vi "pmtProjectorGating2.vi"() -> ()   [LabVIEW 2012]
doc: "I. Description:\nThis example demonstrates how to output a retriggerable waveform using the internal output of a counter for the sample clock.\n\nII. Instructions for Running:\n1. Select the Physical Channel to correspond to where your signal is output on the DAQ device.\n2. Enter the Minimum and Maximum Voltage Ranges\n3. Enter the Counter Channel to generate a pulse train for the sample clock\n4. Select the Clock Source to be the Internal Output of the counter chosen in the previous step. If you cannot see this option, right-click on the control, choose I/O Name Filtering …, and select \"Include Advanced Terminals\" \n5. Select the Trigger Source to correspond to the terminal on which the trigger will be received\n6. Select the Trigger Edge to be rising or falling\n7. Specify the Desired Frequency of the output Waveform\n8. Enter the Waveform Information. See the documentation of the Waveform Buffer Generation SubVI for information on each parameter.\n\nIII. Block Diagram Steps:\nSteps: \n1. Create an Analog Output Voltage channel and a Counter Output Frequency channel.\n2. Use the Waveform Buffer subVI to create the waveform. \n3. Call the DAQmx Timing (Implicit) VI which sets the sample clock rate based on the frequency of the pulse train, and set the sample mode to finite. The number of Sample per Buffer corresponds to the number of samples per channel the counter output channel will produce. Set the DAQmx Timing (Sample Clock) VI to use the Internal Output of the counter as its Clock Source and set the sample mode to continuous.\n4. Call the DAQmx Start Trigger VI to set the Source and Trigger Edge. \n5. Write the waveform to the output buffer.\n6. Use the DAQmx Trigger Property Node to allow retriggerable operation for the counter.\n7. Call the Start VI for the Analog Output task.\n8. Call the Start VI for the Counter Output task.\n9. Loop continuously until the user presses the Stop button. Check for errors every 100 ms using the Is Task Done? VI\n10. Clear the Task\n11. Use the popup dialog box to display an error or warning if any.\n\nIV. I/O Connections Overview:\nMake sure your signal output terminal matches the Physical Channel I/O Control. For further connection information, refer to your hardware reference manual."
uses:
  <vilib>/Utility/error.llb/DialogType.ctl
  <vilib>/DAQmx/write.llb/DAQmx Write (Digital 1D Wfm NChan NSamp).vi
  <vilib>/DAQmx/write.llb/DAQmx Write (Digital 1D Bool NChan 1Samp 1Line).vi
  <vilib>/DAQmx/create/channels.llb/DAQmx Create Channel (DO-Digital Output).vi
  <vilib>/DAQmx/configure/timing.llb/DAQmx Timing (Sample Clock).vi
  <vilib>/DAQmx/create/channels.llb/DAQmx Create Channel (CO-Pulse Generation-Frequency).vi
  <vilib>/DAQmx/configure/timing.llb/DAQmx Timing (Implicit).vi
  <vilib>/Waveform/DWDTOps.llb/DWDT Analog to Digital.vi
  <vilib>/DAQmx/configure/trigger.llb/DAQmx Start Trigger (Digital Edge).vi
  <vilib>/Waveform/DWDTOps.llb/DWDT Uncompress Digital.vi
  <vilib>/DAQmx/miscellaneous.llb/DAQmx Fill In Error Info.vi
  <resource>/objmgr/daqmx.rc
panel:
  in  "refreshing":bool
  in  "Tab":enum32{"Timing", "Channels", "Extras"}(tab)
  in  "Proj. Initial delay [us]":i32=2
  in  "PMT Initial delay [us]":i32
  in  "PMT Pulse duration [us]":i32=60
  in  "PMT Pulse spacing [us]":i32=1
  in  "Proj. Pulse duration [us]":i32=30
  in  "Proj. Pulse spacing [us]":i32=29
  out "Frame counting (VRE14.vi)":tag="Dev2/ctr2"
  in  "Counter for external trigger":tag="Dev2/ctr1"
  out "Scanning state (RS syncH)":tag="Dev2/AI0"
  in  "PMT gating":tag="Dev2/port0/line0"
  in  "projector gating":tag="Dev2/port0/line2"
  in  "Clock":tag="/Dev2/Ctr3InternalOutput"
  in  "Counter for timing DO":tag="Dev2/ctr3"
  in  "Trigger for gating (RS or Ctr1)":tag="/Dev2/PFI3"
  in  "stop":bool
  in  "Help":bool caption="stop"
  # "This code requires resonant scanner being powered."
  # "Timing"
  # "2P gating"
  # "non-2P gating"
  # "Other"
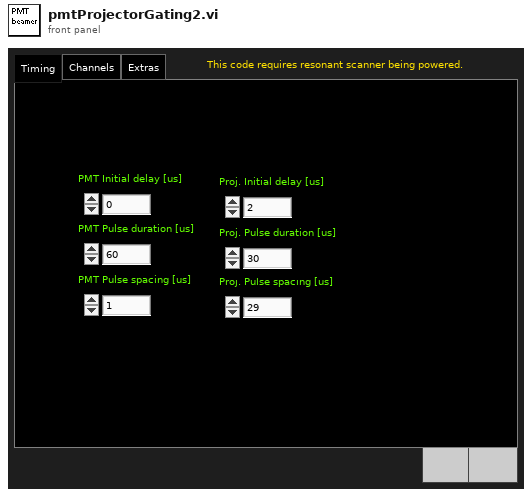
[diagram p1: front panel]
types:
  T1 = typedef "DialogType.ctl" = u16
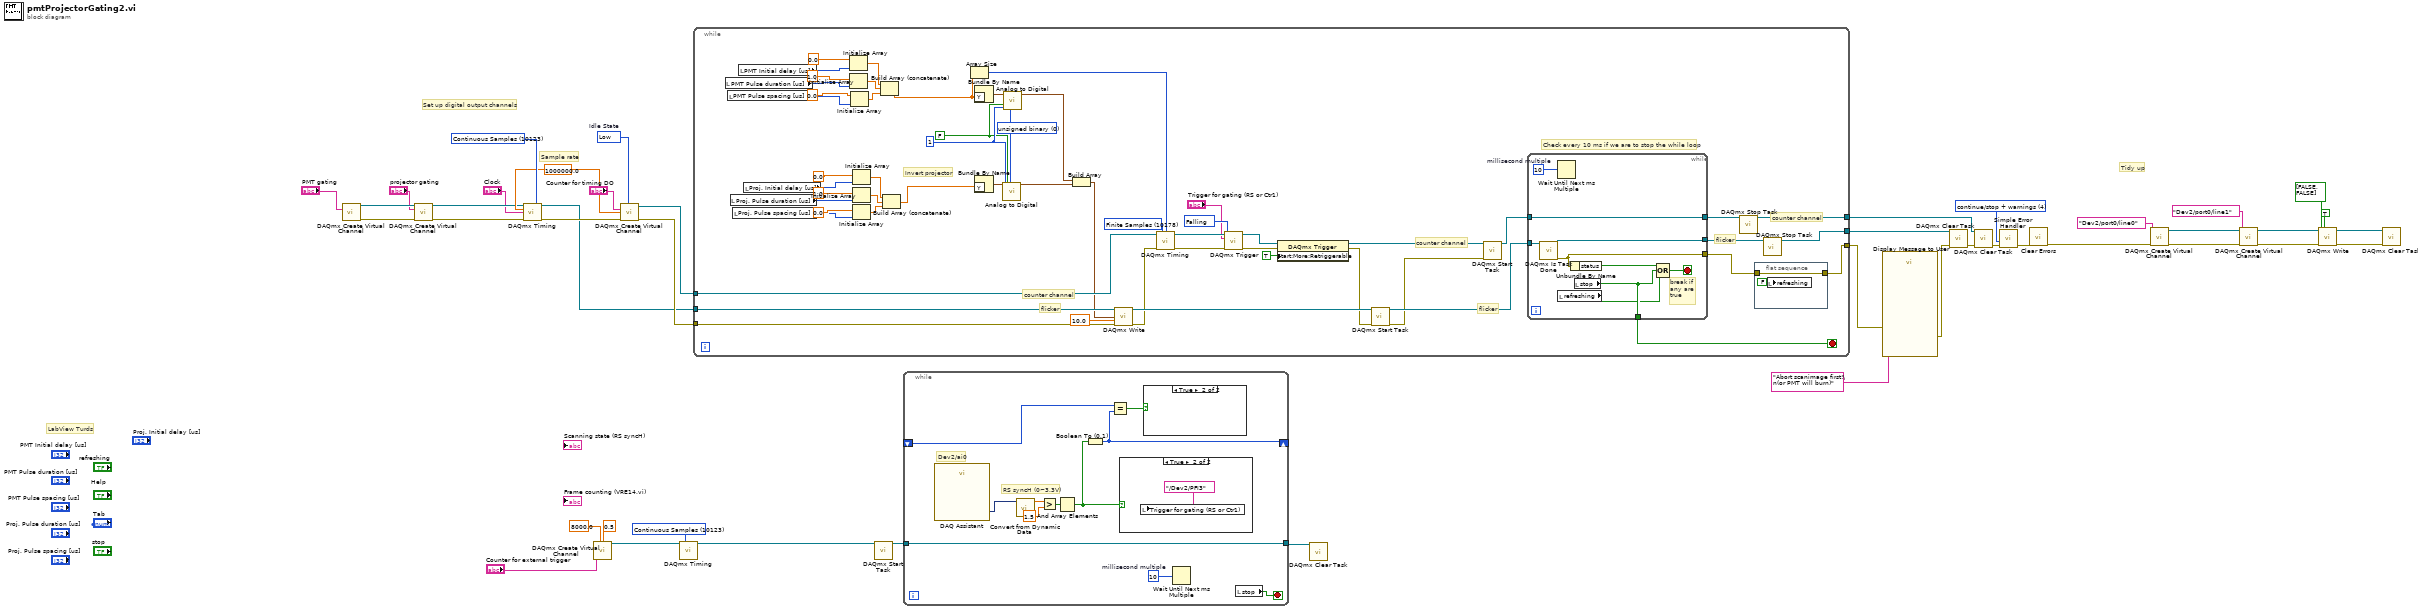
[diagram p0: block diagram]
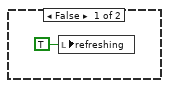
[diagram p2: hidden frame]
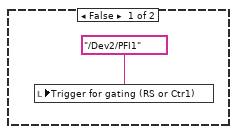
[diagram p3: hidden frame]
diagram:
  w9 = 10123 items=["Finite Samples"=10178, "Continuous Samples"=10123, "Hardware Timed Single Point"=12522] ("sample mode")
  w22 = T1 4 items=["no dialog", "OK message", "continue or stop message", "OK message + warnings", "continue/stop + warnings"] ("type of dialog (OK msg:1)")
  w27 = 1000000.0 ("frequency")
  w30 = 10214 items=["High"=10192, "Low"=10214]  # Idle State
  w32 = 10123 items=["Finite Samples"=10178, "Continuous Samples"=10123] ("sample mode")
  # "Tidy up"
  # "Set up digital output channels"
  # "Sample rate"
  # "LabView Turds"
  n1 = call-poly <vilib>:"DAQmx Create Virtual Channel.vi"("lines"="PMT gating") -> ("task out"=w34:refnum<k21>, "error out"=w33:errorcluster)  [unwired: 13 in]
  n2 = call-poly <vilib>:"DAQmx Create Virtual Channel.vi"("task in"=w34, "lines"="projector gating", "error in"=w33) -> ("task out"=w26:refnum<k21>, "error out"=w31:errorcluster)  [unwired: 11 in]
  n3 = call-poly <vilib>:"DAQmx Timing.vi"("task/channels in"=w26, "sample mode"=w32, "rate"=w27, "source"="Clock", "error in"=w31) -> ("task out"=w18:refnum<k21>, "error out"=w29:errorcluster)  [unwired: 9 in]
  n4 = call-poly <vilib>:"DAQmx Create Virtual Channel.vi"("frequency"=8000.0, "duty cycle"=0.5, "counter"="Counter for external trigger") -> ("task out"=w8:refnum<k21>)  [unwired: 11 in, 1 out]
  n5 = call-poly <vilib>:"DAQmx Create Virtual Channel.vi"("frequency"=w27, "counter"="Counter for timing DO", "error in"=w29, "idle state"=w30) -> ("task out"=w25:refnum<k21>, "error out"=w28:errorcluster)  [unwired: 10 in]
  n6 = call-poly <vilib>:"DAQmx Timing.vi"("task/channels in"=w8, "sample mode"=w9) -> ("task out"=w4:refnum<k21>)  [unwired: 12 in, 1 out]
  n7 = while {
    tunnel: w18 -> [w73]
    tunnel: w28 -> [w72]
    tunnel: w25 -> [w66]
    tunnel: [w61] -> w21
    tunnel: [w60] -> w20
    tunnel: [w64] -> w3
    stop <- w98 stop-if-true
    w46 = 10171 items=["Rising"=10280, "Falling"=10171] ("edge")
    w75 = 1 ("resolution (16 bit)")
    w76 = u16 0 items=["unsigned binary", "offset binary", "2's complement"] ("data format (offset binary)")
    w74 = FALSE ("compress digital (T)")
    w95 = 10178 items=["Finite Samples"=10178, "Continuous Samples"=10123] ("sample mode")
    # "Check every 10 ms if we are to stop the while loop"
    # "counter channel"
    # "counter channel"
    # "flicker"
    # "flicker"
    # "flicker"
    # "counter channel"
    # "Invert projector"
    n8 = local read "PMT Pulse duration [us]"() -> (w82:i32)
    n9 = local read "PMT Pulse spacing [us]"() -> (w81:i32)
    n10 = local read "Proj. Pulse duration [us]"() -> (w49:i32)
    n11 = local read "Proj. Pulse spacing [us]"() -> (w47:i32)
    n12 = local read "PMT Initial delay [us]"() -> (w83:i32)
    n13 = local read "Proj. Initial delay [us]"() -> (w51:i32)
    n14 = Initialize Array(0.0 ("element"), w83) -> (w87:dbl[])
    n15 = Initialize Array(1.0 ("element"), w82) -> (w85:dbl[])
    n16 = Initialize Array(0.0 ("element"), w81) -> (w88:dbl[])
    n17 = Initialize Array(0.0 ("element"), w51) -> (w57:dbl[])
    n18 = Initialize Array(1.0 ("element"), w49) -> (w58:dbl[])
    n19 = Initialize Array(0.0 ("element"), w47) -> (w56:dbl[])
    n20 = Build Array (concatenate)(w87, w85, w88) -> (w80:dbl[])
    n21 = Build Array (concatenate)(w57, w58, w56) -> (w45:dbl[])
    n22 = Array Size(array=w80) -> (size(s)=w86:i32)
    n23 = Bundle By Name("Y"=w80) -> (w84:waveform(dbl))  [unwired: 1 in]
    n24 = Bundle By Name("Y"=w45) -> (w78:waveform(dbl))  [unwired: 1 in]
    n25 = call-poly <vilib>:"Analog to Digital.vi"("data format (offset binary)"=w76, "compress digital (T)"=w74, "resolution (16 bit)"=w75, "analog waveform"=w78) -> ("digital waveform"=w77:digitalwaveform)  [unwired: 4 in, 3 out]
    n26 = call-poly <vilib>:"Analog to Digital.vi"("data format (offset binary)"=w76, "compress digital (T)"=w74, "resolution (16 bit)"=w75, "analog waveform"=w84) -> ("digital waveform"=w79:digitalwaveform)  [unwired: 4 in, 3 out]
    n27 = Build Array(w79, w77) -> (w59:digitalwaveform[])
    n28 = call-poly <vilib>:"DAQmx Write.vi"("task/channels in"=w73, "data"=w59, "timeout"=10.0 ("Wirite Timeout"), "error in"=w72) -> ("task out"=w89:refnum<k21>, "error out"=w71:errorcluster)  [unwired: 9 in, 1 out]
    n29 = call-poly <vilib>:"DAQmx Timing.vi"("task/channels in"=w66, "sample mode"=w95, "samples per channel"=w86, "error in"=w71) -> ("task out"=w94:refnum<k21>, "error out"=w70:errorcluster)  [unwired: 10 in]
    n30 = call-poly <vilib>:"DAQmx Trigger.vi"("task/channels in"=w94, "source"="Trigger for gating (RS or Ctr1)", "edge"=w46, "error in"=w70) -> ("task out"=w92:refnum<k21>, "error out"=w69:errorcluster)  [unwired: 10 in]
    n31 = property class="DAQmx Trigger"(reference=w92, error in=w69, "Start:More:Retriggerable"=TRUE) -> (reference out=w91:refnum<k21>, error out=w68:errorcluster)
    n32 = call <vilib>:"DAQmx Start Task.vi"("task/channels in"=w89, "error in"=w68) -> ("task out"=w96:refnum<k21>, "error out"=w67:errorcluster)  [unwired: 12 in]
    n33 = call <vilib>:"DAQmx Start Task.vi"("task/channels in"=w91, "error in"=w67) -> ("task out"=w90:refnum<k21>)  [unwired: 12 in, 1 out]
    n34 = while {
      tunnel: w96 -> [w109]
      tunnel: [w108] -> w62
      tunnel: [w107] -> w65
      tunnel: w90 -> [w103]
      tunnel: [w103] -> w63
      tunnel: [w102] -> w98
      stop <- w105 stop-if-true
      w106 = u32 10  # millisecond multiple
      # "break if\nany are \ntrue"
      n35 = call <vilib>:"DAQmx Is Task Done.vi"("task/channels in"=w109) -> ("task out"=w108:refnum<k21>, "error out"=w107:errorcluster)  [unwired: 12 in, 1 out]
      n36 = Wait Until Next ms Multiple(millisecond multiple=w106) -> ()  [unwired: 1 out]
      n37 = local read "refreshing"() -> (w101:bool)
      n38 = Unbundle By Name(w107) -> ("status"=w104:bool)
      n39 = local read "stop"() -> (w102:bool)
      n40 = Compound Arithmetic op=OR(w104, w102, w101) -> (w105:bool)
    }
    n41 = call <vilib>:"DAQmx Stop Task.vi"("task/channels in"=w63) -> ("task out"=w61:refnum<k21>)  [unwired: 13 in, 1 out]
    n42 = flat-sequence {
      tunnel: w65 -> [w100]
      tunnel: [w100] -> w64
      frame #0 {
        n43 = local write "refreshing"(FALSE ("Boolean")) -> ()
      }
    }
    n44 = call <vilib>:"DAQmx Stop Task.vi"("task/channels in"=w62) -> ("task out"=w60:refnum<k21>)  [unwired: 13 in, 1 out]
  }
  n45 = call <vilib>:"DAQmx Start Task.vi"("task/channels in"=w4) -> ("task out"=w6:refnum<k21>)  [unwired: 13 in, 1 out]
  n46 = while {
    tunnel: w6 -> [w116]
    tunnel: [w116] -> w5
    shift-right: [w110] -> _
    shift-left: _ -> [w113]
    stop <- w117 stop-if-true
    w115 = u32 10  # millisecond multiple
    # "RS syncH (0~3.3V)"
    # "Dev2/ai0"
    n47 = call "DAQ Assistant"() -> ("data"=w111:dynamicdata)  [unwired: 17 in, 2 out]
    n48 = call "Convert from Dynamic Data"("Dynamic Data Type"=w111) -> ("Array"=w120:dbl[])  [unwired: 3 in]
    n49 = Greater?(x=w120, y=1.5) -> (0:w118:bool[])
    n50 = And Array Elements(Boolean array=w118) -> (logical AND=w114:bool)
    n51 = Boolean To (0,1)(Boolean=w114) -> (0, 1=w110:i16)
    n52 = Equal?(x=w113, y=w110) -> (x = y?=w112:bool)
    n53 = case shown="True" w114 {
      frame False {
        n54 = local write "Trigger for gating (RS or Ctr1)"(tag "/Dev2/PFI1" ("Trigger for gating 2")) -> ()
      }
      frame True {
        n55 = local write "Trigger for gating (RS or Ctr1)"(tag "/Dev2/PFI3" ("Trigger for gating")) -> ()
      }
    }
    n56 = case shown="True" w112 {
      frame False {
        n57 = local write "refreshing"(TRUE ("refreshing")) -> ()
      }
      frame True {
      }
    }
    n58 = Wait Until Next ms Multiple(millisecond multiple=w115) -> ()  [unwired: 1 out]
    n59 = local read "stop"() -> (w117:bool)
  }
  n60 = call <vilib>:"DAQmx Clear Task.vi"("task in"=w5) -> ()  [unwired: 14 in, 1 out]
  n61 = call "Display Message to User"("error in (no error)"=w3, "Message"="Abort scanimage first!\n(or PMT will burn)") -> ("error out"=w2:errorcluster)  [unwired: 8 in, 1 out]
  n62 = call <vilib>:"DAQmx Clear Task.vi"("task in"=w20, "error in"=w2) -> ("error out"=w23:errorcluster)  [unwired: 13 in]
  n63 = call <vilib>:"DAQmx Clear Task.vi"("task in"=w21, "error in"=w23) -> ("error out"=w24:errorcluster)  [unwired: 13 in]
  n64 = call <vilib>:"Simple Error Handler.vi"("type of dialog (OK msg:1)"=w22, "error in (no error)"=w24) -> ("error out"=w19:errorcluster)  [unwired: 3 in, 4 out]
  n65 = call <vilib>:"Clear Errors.vi"("error in (no error)"=w19) -> ("error out"=w38:errorcluster)  [unwired: 6 in]
  n66 = call-poly <vilib>:"DAQmx Create Virtual Channel.vi"("lines"=tag "Dev2/port0/line0", "error in"=w38) -> ("task out"=w42:refnum<k21>, "error out"=w43:errorcluster)  [unwired: 12 in]
  n67 = call-poly <vilib>:"DAQmx Create Virtual Channel.vi"("task in"=w42, "lines"=tag "Dev2/port0/line1", "error in"=w43) -> ("task out"=w41:refnum<k21>, "error out"=w40:errorcluster)  [unwired: 11 in]
  n68 = call-poly <vilib>:"DAQmx Write.vi"("task/channels in"=w41, "auto start"=TRUE, "data"=bool[] [FALSE, FALSE], "error in"=w40) -> ("task out"=w36:refnum<k21>, "error out"=w37:errorcluster)  [unwired: 9 in, 1 out]
  n69 = call <vilib>:"DAQmx Clear Task.vi"("task in"=w36, "error in"=w37) -> ()  [unwired: 13 in, 1 out]
